vi "FTW-Endpoint-Receive.vi"(0 "FTW Endpoint":refnum<class "FTW-Endpoint-TCP.lvclass">, 5 "Timeout":i32 format="%dmsec", 11 "error in":errorcluster) -> (4 "FTW Endpoint out":refnum<class "FTW-Endpoint-TCP.lvclass">, 6 "Message Header":string, 8 "Message Body":string, 10 "Timed out?":bool, 15 "error out":errorcluster)   [LabVIEW 2013, in "FTW-Endpoint-TCP.lvclass"]
uses:
  FTW-Endpoint-TCP.lvclass
panel:
  # "Inputs"
  # "Outputs"
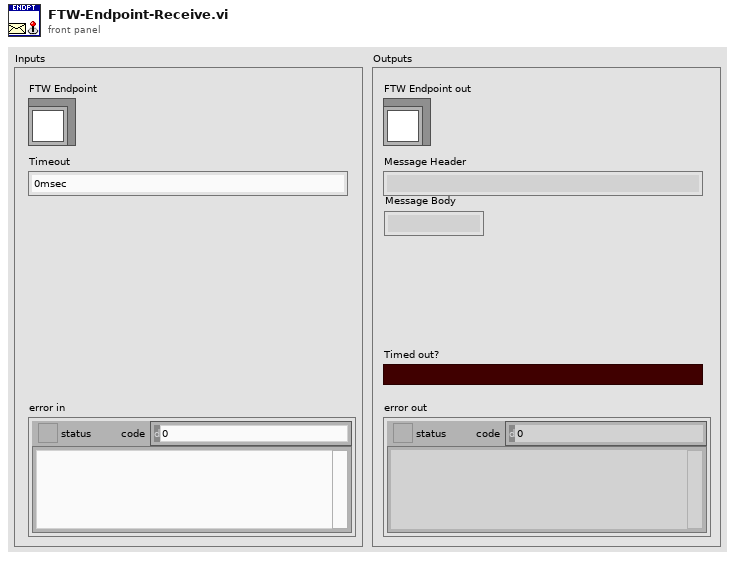
[diagram p1: front panel]
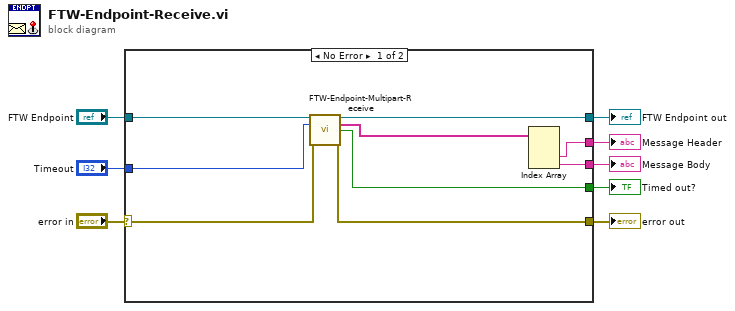
[diagram p0: block diagram]
diagram:
  n1 = case shown="No Error" "error in" {
    selector: "error in" -> [w12 w19]
    tunnel: [w11 w19] -> w8
    tunnel: [w9 w18] -> w6
    tunnel: "FTW Endpoint" -> [w15 w18]
    tunnel: [w10 _] -> w4
    tunnel: "Timeout" -> [w13 _]
    tunnel: [w17 _] -> w2
    tunnel: [w16 _] -> w1
    frame No Error {
      n2 = call-dynamic "FTW-Endpoint-Multipart-Receive.vi"("FTW Endpoint"=w15, "Timeout"=w13, "error in"=w12) -> ("FTW Endpoint out"=w9:refnum<class "FTW-Endpoint-TCP.lvclass">, "Message Received"=w14:string[], "Timed out?"=w10:bool, "error out"=w11:errorcluster)  [unwired: 9 in]
      n3 = Index Array(array=w14) -> (element #2=w17:string, element #3=w16:string)  [unwired: 3 in, 1 out]
    }
    frame Error {
    }
  }
  "error out" <- w8
  "FTW Endpoint out" <- w6
  "Timed out?" <- w4
  "Message Header" <- w2
  "Message Body" <- w1
